vi "init_motorsystem.vi"(7 "dimension names":string[](array[string]), 8 "error in (no error)":errorcluster caption="错误输入（无错误）", 9 "CAN node IDs":u32[](array[numeric]), 10 "device index":u32, 11 "MotorSystem 输入":refnum<class "MotorSystem.lvclass">) -> (0 "error out":errorcluster caption="错误输出", 3 "MotorSystem 输出":refnum<class "MotorSystem.lvclass">)   [LabVIEW 2016, in "MotionControl_UFO_3DOF.lvlib" / "MotorSystem.lvclass"]
uses:
  <userlib>/MotionControl_UFO_3DOF/MotorSystem/MotorSystem.lvclass
  <userlib>/MotionControl_UFO_3DOF/MotorSystem/MotorSystem.lvclass/MotorSystem.ctl
  <userlib>/MotionControl_UFO_3DOF/OneMotion/OneMotion.lvclass
  <userlib>/MotionControl_UFO_3DOF/MotorSystem/MotionCluster.ctl
  <userlib>/MotionControl_UFO_3DOF/OneMotion/OneMotion.lvclass/OneMotion.ctl
  <userlib>/MotionControl_UFO_3DOF/OneMotion/set_fault.vi
  <vilib>/Utility/config.llb/NI_LVConfig.lvlib
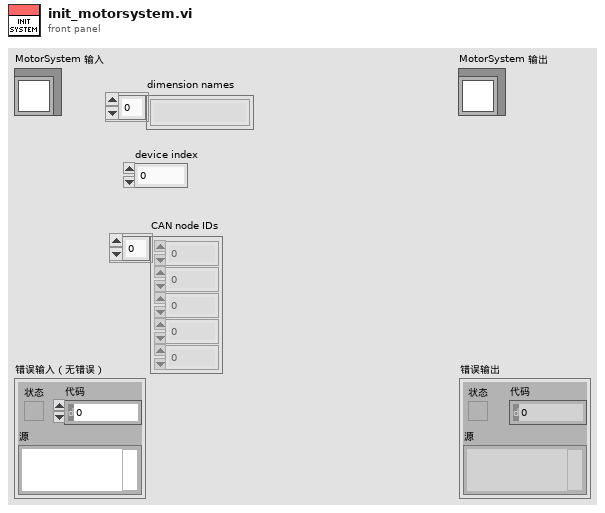
[diagram p1: front panel]
types:
  T1 = typedef "MotionControl_UFO_3DOF.lvlib/MotorSystem.lvclass/MotionCluster.ctl" = cluster{"OneMotion.lvclass":refnum<class "OneMotion.lvclass">, "connected?":bool, "default enabled?":bool, "enabled?":bool}
  T2 = typedef "NI_LVConfig.lvlib/Config Data RefNum.ctl" = refnum<k1>
  T3 = typedef "MotionControl_UFO_3DOF.lvlib/MotorSystem.lvclass/SavedPosCluster.ctl" = cluster{"name":string, "command list":T4}
  T4 = typedef "MotionControl_UFO_3DOF.lvlib/MotorSystem.lvclass/CommandList.ctl" = cluster{"cmd":T5, "cmd info":T6[]}[]
  T5 = typedef "MotionControl_UFO_3DOF.lvlib/MotorSystem.lvclass/cmd_system.ctl" = enum16{"NONE", "MOVE_SYSTEM", "WAIT_UNTIL_MOVE_DONE", "EXIT", "WAIT_UNTIL_SELECTED_MOVE_DONE", "WAIT_A_TIME"}
  T6 = typedef "MotionControl_UFO_3DOF.lvlib/MotorSystem.lvclass/SavedDimensionCluster.ctl" = cluster{"dimension name":string, "pos":dbl, "unit mode":T7, "unit conversion ratio":dbl}
  T7 = typedef "MotionControl_UFO_3DOF.lvlib/OneMotion.lvclass/unit mode.ctl" = enum16{"motor (pulse)", "linear (mm) or radial (degree)"}
  T8 = cluster{"array for a soft limit":cluster{"dim name":string, "soft limit":cluster{"min":dbl, "max":dbl}}[]}[]
  T9 = cluster{"complete dimension names[0]":string, "complete dimension names[1]":string, "complete dimension names[2]":string}
  T10 = cluster{"complete dimension names":string[], "dimension names cluster ":cluster{"name 1":string, "name 2":string, "name 3":string}}
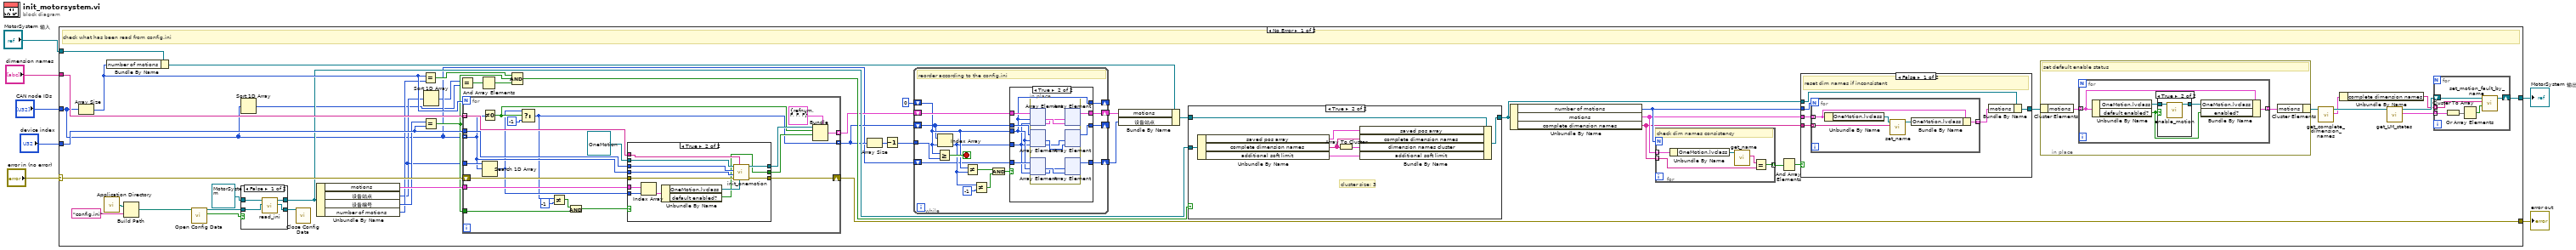
[diagram p0: block diagram]
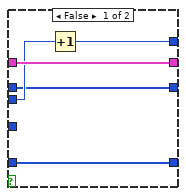
[diagram p2: hidden frame]
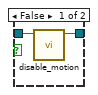
[diagram p3: hidden frame]
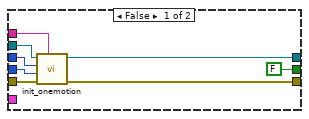
[diagram p7: hidden frame]
diagram:
  n1 = case shown="No Error" "error in (no error)" {
    selector: "error in (no error)" -> [w55 w180]
    tunnel: [w53 w180] -> w6
    tunnel: [w23 w179] -> w4
    tunnel: "MotorSystem 输入" -> [w54 w179]
    tunnel: "CAN node IDs" -> [w12 _]
    tunnel: "device index" -> [w45 _]
    tunnel: "dimension names" -> [w52 _]
    frame No Error {
      # "check what has been read from config.ini"
      n2 = Array Size(array=w12) -> (size(s)=w42:i32)
      n3 = call <vilib>:"Application Directory.vi"() -> ("Application Directory"=w51:path)
      n4 = Bundle By Name(cluster=w54, "number of motions"=w42) -> (w56:refnum<class "MotorSystem.lvclass">)
      n5 = Build Path(base path=w51, name or relative path="config.ini" ("名称或相对路径")) -> (appended path=w46:path)
      n6 = call <vilib>:"Open Config Data.vi"("configuration file path"=w46) -> ("file created?"=w31:bool, "refnum"=w49:T2)  [unwired: 8 in, 1 out]
      n7 = Sort 1D Array(array=w12) -> (sorted array=w8:u32[])
      n8 = case shown="False" w31 {
        tunnel: w49 -> [w111 w112]
        tunnel: [w110 w112] -> w48
        tunnel: refnum<class "MotorSystem.lvclass"> refnum ("MotorSystem.lvclass") -> [w109 w113]
        tunnel: [w108 w113] -> w37
        frame False {
          n9 = call-dynamic "read_ini.vi"("file ref in"=w111, "MotorSystem 输入"=w109) -> ("file ref out"=w110:T2, "MotorSystem 输出"=w108:refnum<class "MotorSystem.lvclass">)  [unwired: 7 in, 1 out]
        }
        frame True {
        }
      }
      n10 = call <vilib>:"Close Config Data.vi"("refnum"=w48) -> ()  [unwired: 9 in, 2 out]
      n11 = Unbundle By Name(w37) -> ("motions"=w44:T1[], "设备站点"=w13:u32[], "设备编号"=w22:u32, "number of motions"=w21:i32)
      n12 = Equal?(x=w42, y=w21) -> (x = y?=w40:bool)
      n13 = Equal?(x=w22, y=w45) -> (x = y?=w41:bool)
      n14 = Sort 1D Array(array=w13) -> (sorted array=w9:u32[])
      n15 = Equal?(x=w9, y=w8) -> (x = y?=w43:bool[])
      n16 = for {
        N: w42 -> [_]
        tunnel: w12 -> [w146] mode=indexing
        tunnel: [w157] -> w18 mode=indexing
        shift-right: [w147] -> w53
        shift-left: w55 -> [w148]
        tunnel: w45 -> [w149]
        tunnel: w52 -> [w150] mode=indexing
        tunnel: w41 -> [w145]
        tunnel: w13 -> [w156]
        tunnel: w44 -> [w154]
        tunnel: [w139] -> w16 mode=indexing
        n17 = Not Equal To 0?(x=w146) -> (x != 0?=w142:bool)
        n18 = Search 1D Array(1D array=w156, element=w146) -> (index of element=w140:i32)  [unwired: 1 in]
        n19 = Select(t=w140, s=w142, f=-1) -> (s? t:f=w139:i32)
        n20 = Not Equal?(x=w139, y=-1) -> (x != y?=w144:bool)
        n21 = And(x=w144, y=w145) -> (x .and. y?=w143:bool)
        n22 = case shown="True" w143 {
          tunnel: w154 -> [_ w178]
          tunnel: w140 -> [_ w177]
          tunnel: [w164 w169] -> w153
          tunnel: [FALSE ("enabled?") w167] -> w152
          tunnel: refnum<class "OneMotion.lvclass"> refnum ("OneMotion.lvclass") -> [w165 w175]
          tunnel: w150 -> [w159 w174]
          tunnel: w149 -> [w162 w173]
          tunnel: w146 -> [w163 w172]
          tunnel: w148 -> [w161 w171]
          tunnel: [w160 w170] -> w147
          frame False {
            n23 = call <userlib>:"init_onemotion.vi"("dimension name"=w159, "error in (no error)"=w161, "CAN node ID"=w163, "device index"=w162, "OneMotion 输入"=w165) -> ("error out"=w160:errorcluster, "OneMotion 输出"=w164:refnum<class "OneMotion.lvclass">)  [unwired: 5 in]
          }
          frame True {
            n24 = Index Array(array=w178, index=w177) -> (element=w176:T1)
            n25 = Unbundle By Name(w176) -> ("OneMotion.lvclass"=w168:refnum<class "OneMotion.lvclass">, "default enabled?"=w167:bool)
            n26 = call <userlib>:"init_onemotion.vi"("OneMotion from file"=w168, "dimension name"=w174, "error in (no error)"=w171, "CAN node ID"=w172, "device index"=w173, "OneMotion 输入"=w175) -> ("error out"=w170:errorcluster, "OneMotion 输出"=w169:refnum<class "OneMotion.lvclass">)  [unwired: 4 in]
          }
        }
        n27 = Bundle(cluster=T1 {"OneMotion.lvclass"=refnum, "connected?"=FALSE, "default enabled?"=FALSE, "enabled?"=FALSE} ("簇"), "OneMotion.lvclass"=w153, "connected?"=w142, "default enabled?"=w152) -> (w157:T1)  [unwired: 1 in]
      }
      n28 = And Array Elements(Boolean array=w43) -> (logical AND=w39:bool)
      n29 = Compound Arithmetic op=AND(w40, w41, w39) -> (w38:bool)
      n30 = Array Size(array=w16) -> (size(s)=w15:i32)
      n31 = Decrement(x=w15) -> (x-1=w10:i32)
      n32 = while {
        shift-right: [w65] -> _
        shift-left: 0 -> [w62]
        shift-right: [w67] -> w14
        shift-left: w18 -> [w68]
        tunnel: w10 -> [w64]
        shift-right: [w59] -> _
        shift-left: w16 -> [w60]
        shift-right: [w57] -> w11
        shift-left: w12 -> [w58]
        stop <- w63 stop-if-true
        # "reorder according to the config.ini"
        n33 = Greater Or Equal?(x=w62, y=w64) -> (x >= y?=w63:bool)
        n34 = Index Array(array=w60, index=w62) -> (element=w61:i32)
        n35 = Not Equal?(x=w62, y=w61) -> (x != y?=w70:bool)
        n36 = Not Equal?(x=w61, y=-1) -> (x != y?=w69:bool)
        n37 = And(x=w70, y=w69) -> (x .and. y?=w66:bool)
        n38 = case shown="True" w66 {
          tunnel: w68 -> [w76 w84]
          tunnel: w62 -> [w75 w79]
          tunnel: w61 -> [_ w78]
          tunnel: [w76 w83] -> w67
          tunnel: [w74 w79] -> w65
          tunnel: w60 -> [w73 w82]
          tunnel: [w73 w81] -> w59
          tunnel: w58 -> [w72 w80]
          tunnel: [w72 w77] -> w57
          frame False {
            n39 = Increment(x=w75) -> (x+1=w74:i32)
          }
          frame True {
            n40 = in-place {
              n41 = in-place-array #1(w84, w79, w78) -> (w90:T1, w89:T1)
              n42 = in-place-array #2(w82, w79, w78) -> (w88:i32, w87:i32)
              n43 = in-place-array #3(w80, w79, w78) -> (w86:u32, w85:u32)
              n44 = in-place-array #1(w89, w90) -> (w83:T1[])  [unwired: 2 out]
              n45 = in-place-array #2(w87, w88) -> (w81:i32[])  [unwired: 2 out]
              n46 = in-place-array #3(w85, w86) -> (w77:u32[])  [unwired: 2 out]
            }
          }
        }
      }
      n47 = Bundle By Name(cluster=w56, "motions"=w14, "设备站点"=w11) -> (w36:refnum<class "MotorSystem.lvclass">)
      n48 = case shown="True" w38 {
        tunnel: w37 -> [_ w136]
        tunnel: w36 -> [w131 w138]
        tunnel: [w131 w133] -> w32
        frame False {
        }
        frame True {
          # "cluster size: 3"
          n49 = Unbundle By Name(w136) -> ("saved pos array"=w137:T3[], "complete dimension names"=w135:string[], "additional soft limit"=w132:T8)
          n50 = Array To Cluster(array=w135) -> (cluster=w134:T9)
          n51 = Bundle By Name(cluster=w138, "saved pos array"=w137, "complete dimension names"=w135, "dimension names cluster"=w134, "additional soft limit"=w132) -> (w133:refnum<class "MotorSystem.lvclass">)
        }
      }
      n52 = Unbundle By Name(w32) -> ("number of motions"=w33:i32, "motions"=w20:T1[], "complete dimension names"=w19:string[])
      n53 = for {
        N: w33 -> [_]
        tunnel: w20 -> [w130] mode=indexing
        tunnel: w19 -> [w127] mode=indexing
        tunnel: [w126] -> w35 mode=indexing
        # "check dim names consistency"
        n54 = Unbundle By Name(w130) -> ("OneMotion.lvclass"=w129:refnum<class "OneMotion.lvclass">)
        n55 = call-dynamic "get_name.vi"("OneMotion输入"=w129) -> ("name"=w128:string)  [unwired: 8 in, 2 out]
        n56 = Equal?(x=w128, y=w127) -> (x = y?=w126:bool)
      }
      n57 = And Array Elements(Boolean array=w35) -> (logical AND=w34:bool)
      n58 = case shown="False" w34 {
        tunnel: w33 -> [w119 _]
        tunnel: w20 -> [w118 _]
        tunnel: w19 -> [w117 _]
        tunnel: w32 -> [w116 w125]
        tunnel: [w114 w125] -> w30
        frame False {
          # "reset dim names if inconsistent"
          n59 = for {
            N: w119 -> [_]
            tunnel: w118 -> [w122] mode=indexing
            tunnel: w117 -> [w123] mode=indexing
            tunnel: [w120] -> w115 mode=indexing
            n60 = Unbundle By Name(w122) -> ("OneMotion.lvclass"=w124:refnum<class "OneMotion.lvclass">)
            n61 = call-dynamic "set_name.vi"("name"=w123, "OneMotion输入"=w124) -> ("OneMotion输出"=w121:refnum<class "OneMotion.lvclass">)  [unwired: 8 in, 1 out]
            n62 = Bundle By Name(cluster=w122, "OneMotion.lvclass"=w121) -> (w120:T1)
          }
          n63 = Bundle By Name(cluster=w116, "motions"=w115) -> (w114:refnum<class "MotorSystem.lvclass">)
        }
        frame True {
        }
      }
      n64 = in-place {
        # "set default enable status"
        n65 = in-place-cluster #4(w30) -> ("motions"=w98:T1[])
        n66 = for {
          tunnel: w98 -> [w102] mode=indexing
          tunnel: [w99] -> w97 mode=indexing
          n67 = Unbundle By Name(w102) -> ("OneMotion.lvclass"=w103:refnum<class "OneMotion.lvclass">, "default enabled?"=w100:bool)
          n68 = case shown="True" w100 {
            tunnel: w103 -> [w105 w107]
            tunnel: [w104 w106] -> w101
            frame False {
              n69 = call <userlib>:"disable_motion.vi"("OneMotion 输入"=w105) -> ("OneMotion 输出"=w104:refnum<class "OneMotion.lvclass">)  [unwired: 9 in, 1 out]
            }
            frame True {
              n70 = call <userlib>:"enable_motion.vi"("OneMotion 输入"=w107) -> ("OneMotion 输出"=w106:refnum<class "OneMotion.lvclass">)  [unwired: 9 in, 1 out]
            }
          }
          n71 = Bundle By Name(cluster=w102, "OneMotion.lvclass"=w101, "enabled?"=w100) -> (w99:T1)
        }
        n72 = in-place-cluster #4("motions"=w97) -> (w27:refnum<class "MotorSystem.lvclass">)
      }
      n73 = call <userlib>:"get_complete_dimension_names.vi"("MotorSystem输入"=w27) -> ("dimension names"=w25:T10, "MotorSystem输出"=w26:refnum<class "MotorSystem.lvclass">)  [unwired: 8 in, 1 out]
      n74 = Unbundle By Name(w25) -> ("complete dimension names"=w24:string[])
      n75 = call <userlib>:"get_LM_states.vi"("MotorSystem 输入"=w26) -> ("LM states"=w29:cluster{"state -":bool, "state +":bool}[], "MotorSystem 输出"=w28:refnum<class "MotorSystem.lvclass">)  [unwired: 8 in, 1 out]
      n76 = for {
        tunnel: w29 -> [w96] mode=indexing
        shift-right: [w93] -> w23
        shift-left: w28 -> [w94]
        tunnel: w24 -> [w92] mode=indexing
        n77 = Cluster To Array(cluster=w96) -> (array=w95:bool[])
        n78 = Or Array Elements(Boolean array=w95) -> (logical OR=w91:bool)
        n79 = call <userlib>:"set_motion_fault_by_name.vi"("fault?"=w91, "name"=w92, "MotorSystem输入"=w94) -> ("MotorSystem输出"=w93:refnum<class "MotorSystem.lvclass">)  [unwired: 7 in, 1 out]
      }
    }
    frame Error {
    }
  }
  "error out" <- w6
  "MotorSystem 输出" <- w4
